vi "Hardware-HH.vi"(8 "error in (no error)":errorcluster, 11 "DCM-DSI in":refnum<class "DCM-DSI.lvclass">) -> (0 "error out":errorcluster, 3 "DCM-DSI out":refnum<class "DCM-DSI.lvclass">)   [LabVIEW 2016, in "DSI-RT.lvlib"]
uses:
  DSI-RT.lvlib
  Classes/DCM-DSI/DCM-DSI.lvclass
  Classes/DCM-DSI/Read DCM Ref.vi
  Classes/DCM-DSI/Read HH Command.vi
  Classes/DCM-DSI/Write HH Command.vi
  <vilib>/Powertrain Controls/Device Drivers/DCM/Rev0/RT/DCM - RT.lvclass
  <vilib>/Powertrain Controls/Device Drivers/DCM/HH/RT/DCM - RT - HH.lvlib
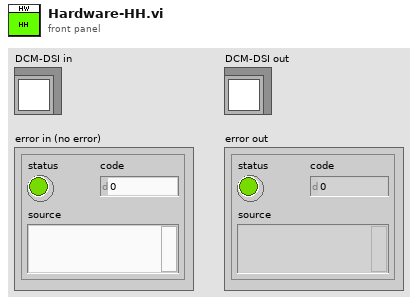
[diagram p1: front panel]
types:
  T1 = typedef "DCM - RT - HH.lvlib/Setup.ctl" = cluster{"Mode":T2, "Digital Input":T3, "Polarity":bool, "Frequency [Hz]":sgl, "Duty Cycle [%]":sgl, "TDC Offset [CAD]":sgl, "Window Start [DBTDC]":sgl, "Window End [DBTDC]":sgl, "Angles":T4[], "Skip Fire":bool, "Skip Fire Index":u8}
  T2 = typedef "DCM - FPGA - HH.lvlib/Mode.ctl" = enum8{"Off", "Direct", "Pulse Width Modulation", "Engine Position Tracking"}
  T3 = typedef "DCM - FPGA.lvlib/Digital Channel.ctl" = enum8{"Unused", "User OS", "Diff IO 1", "Diff IO 2", "Diff IO 3", "Diff IO 4", "Diff IO 5", "Diff IO 6", "Diff IO 7", "Diff IO 8", "Aux 1", "Aux 2", "Aux 3", "Aux 4", "Aux 5", "Aux 6", "Aux 7", "Aux 8", "Aux 9", "Aux 10", "Aux 11", "Aux 12", "Aux 13", "Aux 14", "Aux 15", "Aux 16"}
  T4 = typedef "DCM - RT - HH.lvlib/Angle Control.ctl" = cluster{"Enable":bool, "Location [DBTDC]":sgl, "Duration [s]":sgl}
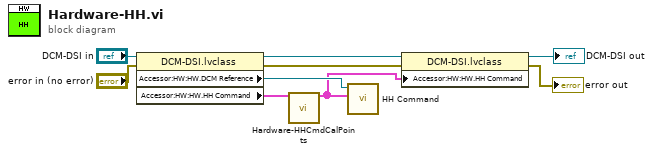
[diagram p0: block diagram]
diagram:
  n1 = property class="DCM-DSI.lvclass"(reference="DCM-DSI in", error in="error in (no error)") -> (reference out=w3:refnum<class "DCM-DSI.lvclass">, error out=w4:errorcluster, "Accessor:HW:HW.DCM Reference"=w5:refnum<class "DCM - RT.lvclass">, "Accessor:HW:HW.HH Command"=w1:T1[])
  n2 = call "Hardware-HHCmdCalPoints.vi"("HH Setup In"=w1) -> ("HH Setup Out"=w2:T1[])  [unwired: 14 in]
  n3 = call <vilib>:"HH Command.vi"("HH Setup"=w2, "DCM Reference"=w5) -> ()  [unwired: 10 in]
  n4 = property class="DCM-DSI.lvclass"(reference=w3, error in=w4, "Accessor:HW:HW.HH Command"=w2) -> (reference out=→"DCM-DSI out":refnum<class "DCM-DSI.lvclass">, error out=→"error out":errorcluster)
